vi "List Class Files From Path Library.vi"(0 "Specified Folder Name":string, 5 "Fixture Or Cal":string, 11 "Error in":errorcluster) -> (4 "Class Files":path[](array[path]), 15 "Error out":errorcluster)   [LabVIEW 2023, in "RFCalAndFixtureCharact.Common.lvlib"]
uses:
  RFCalAndFixtureCharact.Common.lvlib
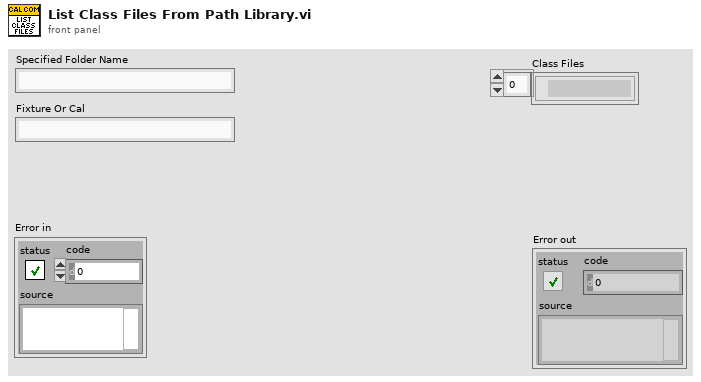
[diagram p1: front panel]
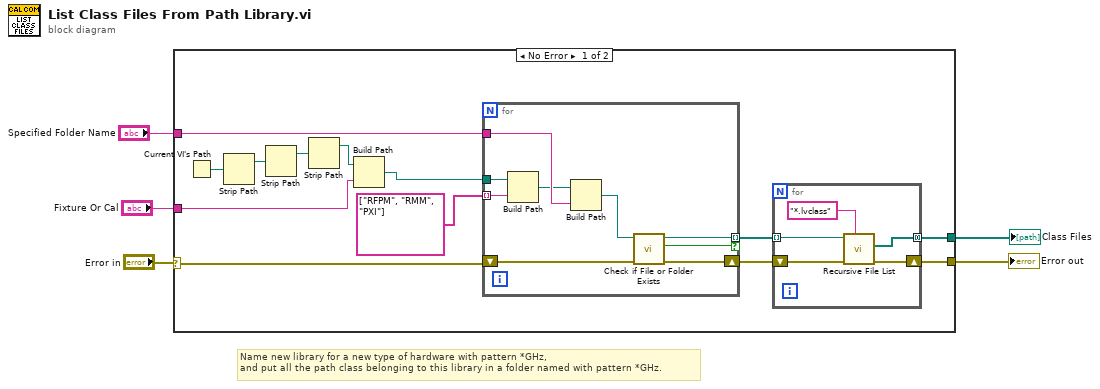
[diagram p0: block diagram]
diagram:
  # "Name new library for a new type of hardware with pattern *GHz, \nand put all the path class belonging to this library in a folder named with pattern *GHz."
  n1 = case shown="No Error" "Error in" {
    selector: "Error in" -> [w7 w33]
    tunnel: "Specified Folder Name" -> [w16 _]
    tunnel: [w14 w33] -> w4
    tunnel: [w13 _] -> w2
    tunnel: "Fixture Or Cal" -> [w8 _]
    frame No Error {
      n2 = Current VI's Path() -> (path=w17:path)
      n3 = Strip Path(path=w17) -> (stripped path=w18:path)  [unwired: 1 out]
      n4 = Strip Path(path=w18) -> (stripped path=w11:path)  [unwired: 1 out]
      n5 = Strip Path(path=w11) -> (stripped path=w10:path)  [unwired: 1 out]
      n6 = Build Path(base path=w10, name or relative path=w8) -> (appended path=w9:path)
      n7 = for {
        tunnel: w16 -> [w32]
        tunnel: string[] ["RFPM", "RMM", "PXI"] ("pattern") -> [w31] mode=indexing
        tunnel: w9 -> [w30]
        tunnel: [w24] -> w15 mode=indexing if=w25
        shift-right: [w26] -> w12
        shift-left: w7 -> [w27]
        n8 = Build Path(base path=w30, name or relative path=w31) -> (appended path=w29:path)
        n9 = Build Path(base path=w29, name or relative path=w32) -> (appended path=w28:path)
        n10 = call <vilib>:"Check if File or Folder Exists.vi"("error in (no error)"=w27, "path"=w28) -> ("error out"=w26:errorcluster, "file or folder exists?"=w25:bool, "dup path"=w24:path)  [unwired: 7 in]
      }
      n11 = for {
        tunnel: [w22] -> w13 mode=concatenating
        tunnel: w15 -> [w21] mode=indexing
        shift-right: [w19] -> w14
        shift-left: w12 -> [w20]
        n12 = call <vilib>:"Recursive File List.vi"("pattern"="*.lvclass", "error in (no error)"=w20, "Folder Path"=w21) -> ("error out"=w19:errorcluster, "All Files in Dir"=w22:path[])  [unwired: 4 in, 3 out]
      }
    }
    frame Error {
    }
  }
  "Error out" <- w4
  "Class Files" <- w2
